vi "CMD_SAVESTATE.vi"(6 "Gantry in":refnum<class "Gantry.lvclass">, 8 "error in (no error)":errorcluster, 10 "Arguments":string[](array[string]), 11 "gScript Interpreter in":refnum<class "gScript Interpreter.lvclass">) -> (0 "error out":errorcluster, 3 "gScript Interpreter out":refnum<class "gScript Interpreter.lvclass">, 4 "Gantry out":refnum<class "Gantry.lvclass">)   [LabVIEW 2017, in "gScript Interpreter.lvclass"]
uses:
  gScript Interpreter.lvclass
  Shared Components/Gantry Class/Gantry.lvclass
  Shared Components/FlexWorktable/FlexWorktable.lvclass
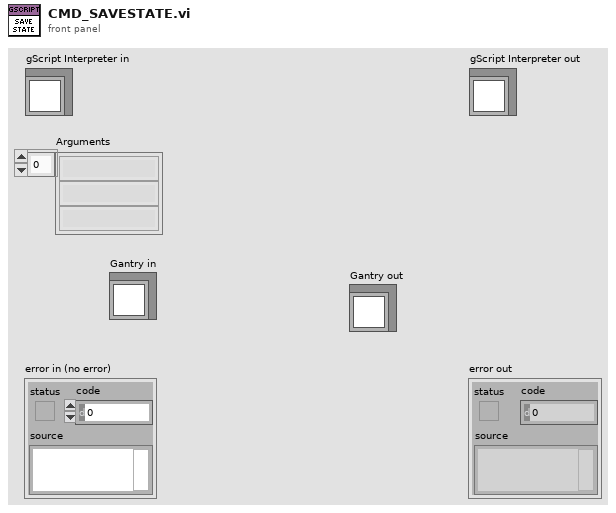
[diagram p1: front panel]
types:
  T1 = enum16{"open", "replace", "create", "open or create", "replace or create", "replace or create with confirmation"}
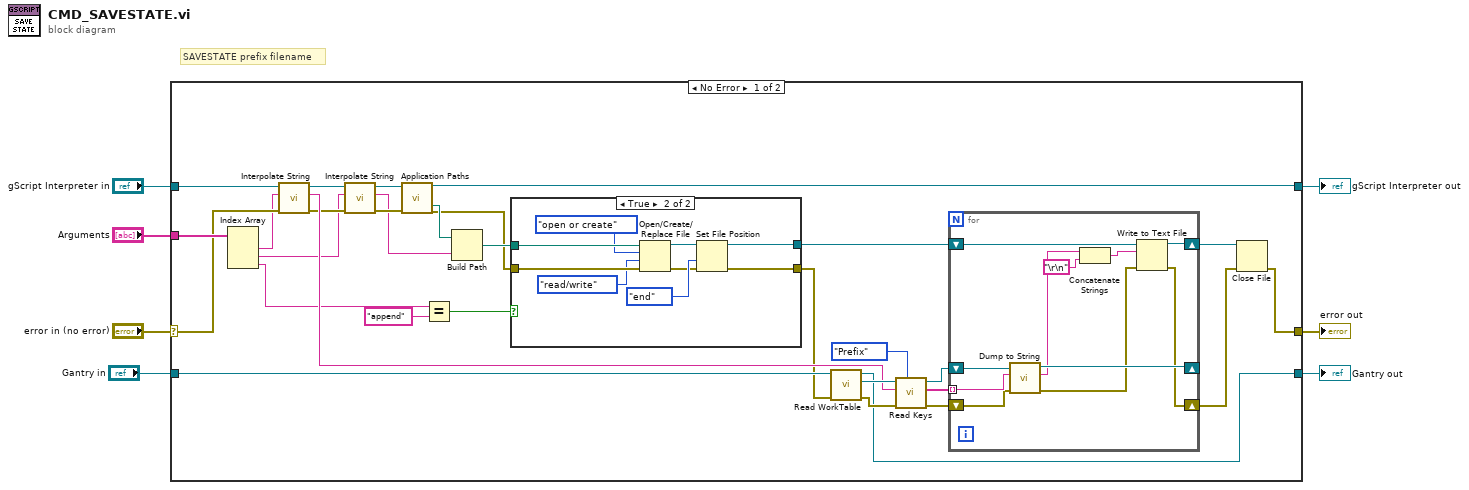
[diagram p0: block diagram]
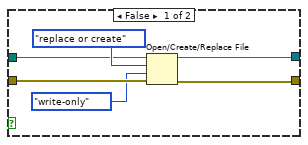
[diagram p2: hidden frame]
diagram:
  # "SAVESTATE prefix filename"
  n1 = case shown="No Error" "error in (no error)" {
    selector: "error in (no error)" -> [w36 w67]
    tunnel: [w8 w67] -> w6
    tunnel: [w15 w66] -> w4
    tunnel: "gScript Interpreter in" -> [w37 w66]
    tunnel: "Arguments" -> [w38 _]
    tunnel: "Gantry in" -> [w34 w65]
    tunnel: [w27 w65] -> w1
    frame No Error {
      n2 = Index Array(array=w38) -> (element #1=w35:string, element #2=w23:string, element #3=w14:string)  [unwired: 3 in]
      n3 = call-dynamic "Interpolate String.vi"("error in (no error)"=w36, "Input String"=w35, "gScript Interpreter in"=w37) -> ("error out"=w24:errorcluster, "Output String"=w26:string, "gScript Interpreter out"=w25:refnum<class "gScript Interpreter.lvclass">)  [unwired: 6 in]
      n4 = call-dynamic "Interpolate String.vi"("error in (no error)"=w24, "Input String"=w23, "gScript Interpreter in"=w25) -> ("error out"=w21:errorcluster, "Output String"=w18:string, "gScript Interpreter out"=w22:refnum<class "gScript Interpreter.lvclass">)  [unwired: 6 in]
      n5 = call "Application Paths.vi"("gScript Interpreter in"=w22, "error in (no error)"=w21) -> ("gScript Interpreter out"=w15:refnum<class "gScript Interpreter.lvclass">, "Logs Path"=w20:path, "error out"=w17:errorcluster)  [unwired: 12 in, 3 out]
      n6 = Equal?(x=w14, y="append") -> (x = y?=w12:bool)
      n7 = Build Path(base path=w20, name or relative path=w18) -> (appended path=w19:path)
      n8 = case shown="True" w12 {
        tunnel: w19 -> [w43 w53]
        tunnel: [w42 w49] -> w11
        tunnel: w17 -> [w41 w52]
        tunnel: [w40 w48] -> w16
        frame False {
          n9 = Open/Create/Replace File(file path (use dialog)=w43, error in=w41, operation (0:open)=T1."replace or create", access (0:read/write)=enum16{"read/write", "read-only", "write-only"}."write-only") -> (refnum out=w42:refnum<file>, error out=w40:errorcluster)  [unwired: 2 in, 1 out]
        }
        frame True {
          n10 = Open/Create/Replace File(file path (use dialog)=w53, error in=w52, operation (0:open)=T1."open or create", access (0:read/write)=enum16{"read/write", "read-only", "write-only"}."read/write") -> (refnum out=w46:refnum<file>, error out=w45:errorcluster)  [unwired: 2 in, 1 out]
          n11 = Set File Position(refnum=w46, from (0:start)=enum16{"start", "end", "current"}."end", error in=w45) -> (refnum out=w49:refnum<file>, error out=w48:errorcluster)  [unwired: 1 in]
        }
      }
      n12 = call-dynamic "Read WorkTable.vi"("error in"=w16, "Gantry Class in"=w34) -> ("error out"=w32:errorcluster, "Worktable"=w33:refnum<class "FlexWorktable.lvclass">, "Gantry Class out"=w27:refnum<class "Gantry.lvclass">)  [unwired: 7 in]
      n13 = call-dynamic "Read Keys.vi"("Prefix/Regex"=enum16{"Prefix", "Regex"}."Prefix", "error in (no error)"=w32, "Selector"=w26, "FlexWorktable in"=w33) -> ("error out"=w28:errorcluster, "Keys"=w31:string[], "FlexWorktable out"=w29:refnum<class "FlexWorktable.lvclass">)  [unwired: 5 in]
      n14 = for {
        tunnel: w31 -> [w63] mode=indexing
        shift-right: [w61] -> _
        shift-left: w29 -> [w64]
        shift-right: [w57] -> w9
        shift-left: w28 -> [w62]
        shift-right: [w59] -> w10
        shift-left: w11 -> [w60]
        n15 = call-dynamic "Dump to String.vi"("error in (no error)"=w62, "Key"=w63, "FlexWorktable in"=w64) -> ("error out"=w58:errorcluster, "Line out"=w56:string, "FlexWorktable out"=w61:refnum<class "FlexWorktable.lvclass">)  [unwired: 6 in]
        n16 = Concatenate Strings(w56, "\r\n") -> (w54:string)
        n17 = Write to Text File(file (use dialog)=w60, text=w54, error in=w58) -> (refnum out=w59:refnum<file>, error out=w57:errorcluster)  [unwired: 1 in, 1 out]
      }
      n18 = Close File(refnum=w10, error in=w9) -> (error out=w8:errorcluster)  [unwired: 1 out]
    }
    frame Error {
    }
  }
  "error out" <- w6
  "gScript Interpreter out" <- w4
  "Gantry out" <- w1
